vi "SDCP SMF Receiver and Transmitter - Tx Table Formatter.vi"(3 "error in (no error)":errorcluster, 4 "Transmit table elements":T1[](array[typedef]), 5 "Table Control":refnum<vi>) -> (0 "error out":errorcluster)   [LabVIEW 2020]
uses:
  Typedefs/SDCP SMF Receiver and Transmitter - Transmit Table Element.ctl
  <vilib>/Utility/miscctls.llb/LVRowAndColumnTypeDef.ctl
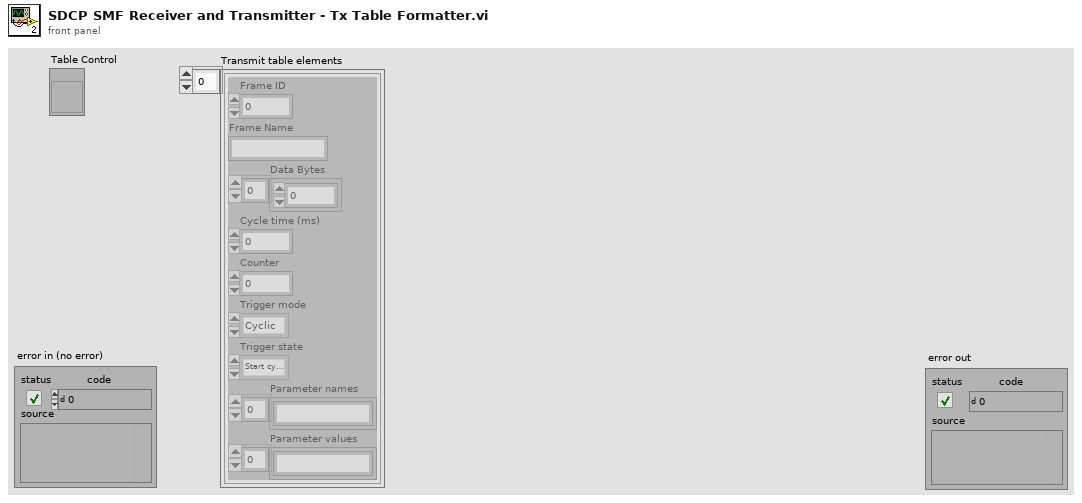
[diagram p1: front panel]
types:
  T1 = typedef "SDCP SMF Receiver and Transmitter - Transmit Table Element.ctl" = cluster{"Frame ID":i32, "Frame Name":string, "Data Bytes":u8[], "Cycle time (ms)":i32, "Counter":i32, "Trigger mode":enum16{"Triggered", "Cyclic"}, "Trigger state":enum16{"Stop cyclic trigger", "Start cyclic trigger", "Stop single trigger", "Start single trigger"}, "Parameter names":string[], "Parameter values":string[]}
  T2 = typedef "LVRowAndColumnTypeDef.ctl" = cluster{"Row":i32, "Column":i32}
  T3 = enum16{"Stop cyclic trigger", "Start cyclic trigger", "Stop single trigger", "Start single trigger"}
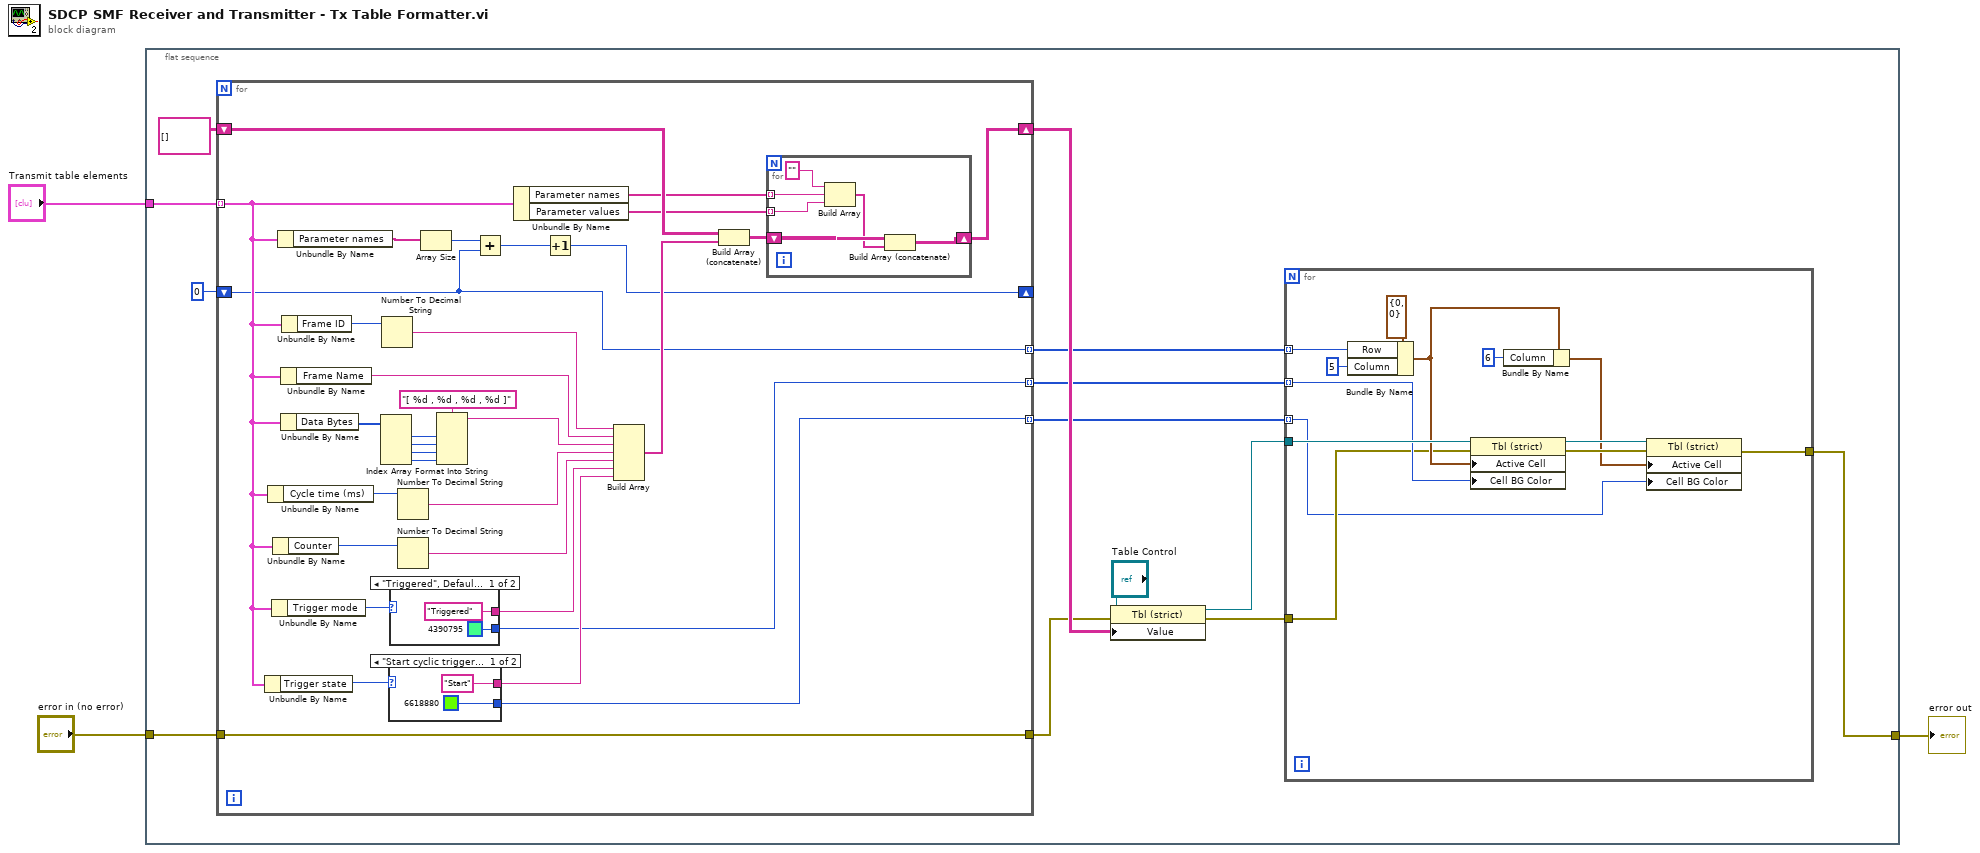
[diagram p0: block diagram]
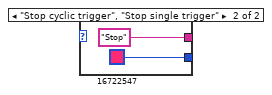
[diagram p2: hidden frame]
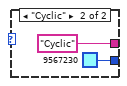
[diagram p3: hidden frame]
diagram:
  n1 = flat-sequence {
    tunnel: "error in (no error)" -> [w16]
    tunnel: "Transmit table elements" -> [w15]
    tunnel: [w5] -> w1
    frame #0 {
      n2 = for {
        tunnel: w16 -> [w62]
        tunnel: [w62] -> w11
        tunnel: w15 -> [w38] mode=indexing
        shift-right: [w30] -> _
        shift-left: 0 -> [w31]
        shift-right: [w35] -> w12
        shift-left: string[][] [] -> [w41]
        tunnel: [w33] -> w9 mode=indexing
        tunnel: [w32] -> w8 mode=indexing
        tunnel: [w31] -> w10 mode=indexing
        n3 = Unbundle By Name(w38) -> ("Trigger state"=w51:T3)
        n4 = Unbundle By Name(w38) -> ("Cycle time (ms)"=w54:i32)
        n5 = Unbundle By Name(w38) -> ("Trigger mode"=w52:enum16{"Triggered", "Cyclic"})
        n6 = Unbundle By Name(w38) -> ("Counter"=w53:i32)
        n7 = Unbundle By Name(w38) -> ("Parameter names"=w43:string[])
        n8 = Unbundle By Name(w38) -> ("Frame Name"=w49:string)
        n9 = Unbundle By Name(w38) -> ("Data Bytes"=w60:u8[])
        n10 = Unbundle By Name(w38) -> ("Frame ID"=w61:i32)
        n11 = Index Array(array=w60) -> (element #1=w58:u8, element #2=w57:u8, element #3=w56:u8, element #4=w55:u8)  [unwired: 4 in]
        n12 = Number To Decimal String(number=w61) -> (decimal integer string=w50:string)  [unwired: 1 in]
        n13 = case shown="\"Start cyclic trigger\", \"Start single trigger\"" w51 {
          tunnel: ["Start" "Stop"] -> w44
          tunnel: [u32 6618880 u32 16722547] -> w32
          frame "Start cyclic trigger", "Start single trigger" {
          }
          frame "Stop cyclic trigger", "Stop single trigger" {
          }
        }
        n14 = case shown="\"Triggered\", Default" w52 {
          tunnel: ["Triggered" "Cyclic"] -> w45
          tunnel: [u32 4390795 u32 9567230] -> w33
          frame "Triggered", Default {
          }
          frame "Cyclic" {
          }
        }
        n15 = Number To Decimal String(number=w54) -> (decimal integer string=w47:string)  [unwired: 1 in]
        n16 = Number To Decimal String(number=w53) -> (decimal integer string=w46:string)  [unwired: 1 in]
        n17 = Array Size(array=w43) -> (size(s)=w42:i32)
        n18 = Format Into String(format string="[ %d , %d , %d , %d ]", w58, w57, w56, w55) -> (resulting string=w48:string)  [unwired: 2 in, 1 out]
        n19 = Add(x=w42, y=w31) -> (x+y=w34:i32)
        n20 = Unbundle By Name(w38) -> ("Parameter names"=w37:string[], "Parameter values"=w36:string[])
        n21 = Increment(x=w34) -> (x+1=w30:i32)
        n22 = Build Array(w50, w49, w48, w47, w46, w45, w44) -> (w40:string[])
        n23 = Build Array (concatenate)(w41, w40) -> (w39:string[][])
        n24 = for {
          shift-right: [w64] -> w35
          shift-left: w39 -> [w66]
          tunnel: w37 -> [w68] mode=indexing
          tunnel: w36 -> [w67] mode=indexing
          n25 = Build Array("" ("element"), w68, w67) -> (w65:string[])
          n26 = Build Array (concatenate)(w66, w65) -> (w64:string[][])
        }
      }
      n27 = property class="Tbl (strict)"(reference="Table Control", error in=w11, "Value"=w12) -> (reference out=w6:refnum<vi>, error out=w7:errorcluster)
      n28 = for {
        tunnel: w10 -> [w27] mode=indexing
        tunnel: w9 -> [w25] mode=indexing
        tunnel: w8 -> [w18] mode=indexing
        tunnel: w7 -> [w22]
        tunnel: w6 -> [w29]
        tunnel: [w17] -> w5
        n29 = Bundle By Name(cluster=T2 {"Row"=0, "Column"=0} ("Active Cell:Active Cell"), "Row"=w27, "Column"=5) -> (w24:T2)
        n30 = property class="Tbl (strict)"(reference=w29, error in=w22, "Active Cell"=w24, "Cell BG Color"=w25) -> (reference out=w20:refnum<vi>, error out=w21:errorcluster)
        n31 = Bundle By Name(cluster=w24, "Column"=6) -> (w19:T2)
        n32 = property class="Tbl (strict)"(reference=w20, error in=w21, "Active Cell"=w19, "Cell BG Color"=w18) -> (error out=w17:errorcluster)  [unwired: 1 out]
      }
    }
  }
  "error out" <- w1
